vi "FPGA Beam Scanning beta.vi"(1 "Detectors":T1, 2 "Image Acquisition Parameters":T2={"Scan Type"=enum."Sample Scanning", "Scan Mode"=enum."XY", "Fast Axis Frequency (Hz)"=100.0, "Image Format"=128, "Line Accumulations"=1, "Frames Per Capture"=1, "Frames Accumulations"=1, "Image Dimension (um)"=[], "Number of Z Steps"=1, "Z Steps Size (um)"=1.0, "Pixel Size (nm)"=[]} {"Z Steps Size (um)" min=0.0; "Number of Z Steps" min=1; "Frames Accumulations" min=1; "Frames Per Capture" min=1; "Line Accumulations" min=1; "Image Format" items=["64 x 64"=64, "128 x 128"=128, "256 x 256"=256, "512 x 512"=512, "1024 x 1024"=1024, "2048 x 2048"=2048]}) -> ()   [LabVIEW 2016]
uses:
  <vilib>/rvi/interface/nirviReadWriteControl/nirviReadWriteControl.xnode
  <vilib>/rvi/interface/nirviMethod/nirviMethod.xnode
  <vilib>/rvi/errors/niLvFpgaMergeErrorWithErrorCode.vi
  <vilib>/rvi/interface/nirviOpenFPGA/nirviOpenFPGA.xnode
  <vilib>/vision/NI_Vision_Development_Module.lvlib
  <vilib>/rvi/interface/nirviCloseFPGA/nirviCloseFPGA.xnode
  <vilib>/vision/Image Controls.llb/IMAQ Image.ctl
  FPGA Bitfiles/MainSTEDFPGAProj_FPGATarget2_BeamScanningCamb_PyGckhW3v70.lvbitx
  FPGA Target VIs/FPGA-7852R/Beam Scanning Cambridge V1.vi
  Type Defs/Image Acquisition Parameters.ctl
  Detectors.ctl
panel:
  in  "line by line":bool
  in  "Adjust Trigger":u16=300
  # "Copyright (C) 2020 Edward S Allgeyer\n\nRedistribution and use in source and binary forms, with or without\nmodification, are permitted provided that the following conditions\nare met:\n\n1. Redistributions of source code must retain the above copyright\n   notice, this list of conditions and the following disclaimer.\n\n2. Redistributions in binary form must reproduce the above copyright\n   notice, this list of conditions and the following disclaimer in\n   the documentation and/or other materials provided with the\n   distribution.\n\n3. Neither the name of the copyright holder nor the names of its\n   contributors may be used to endorse or promote products derived\n   from this software without specific prior written permission.\n\nTHIS SOFTWARE IS PROVIDED BY THE COPYRIGHT HOLDERS AND CONTRIBUTORS\n\"AS IS\" AND ANY EXPRESS OR IMPLIED WARRANTIES, INCLUDING, BUT NOT\nLIMITED TO, THE IMPLIED WARRANTIES OF MERCHANTABILITY AND FITNESS\nFOR A PARTICULAR PURPOSE ARE DISCLAIMED. IN NO EVENT SHALL THE\nCOPYRIGHT HOLDER OR CONTRIBUTORS BE LIABLE FOR ANY DIRECT, INDIRECT,\nINCIDENTAL, SPECIAL, EXEMPLARY, OR CONSEQUENTIAL DAMAGES (INCLUDING,\nBUT NOT LIMITED TO, PROCUREMENT OF SUBSTITUTE GOODS OR SERVICES;\nLOSS OF USE, DATA, OR PROFITS; OR BUSINESS INTERRUPTION) HOWEVER\nCAUSED AND ON ANY THEORY OF LIABILITY, WHETHER IN CONTRACT, STRICT\nLIABILITY, OR TORT (INCLUDING NEGLIGENCE OR OTHERWISE) ARISING IN\nANY WAY OUT OF THE USE OF THIS SOFTWARE, EVEN IF ADVISED OF THE\nPOSSIBILITY OF SUCH DAMAGE."
  # "XY"
  # "Z"
  # "Length"
  # "Height"
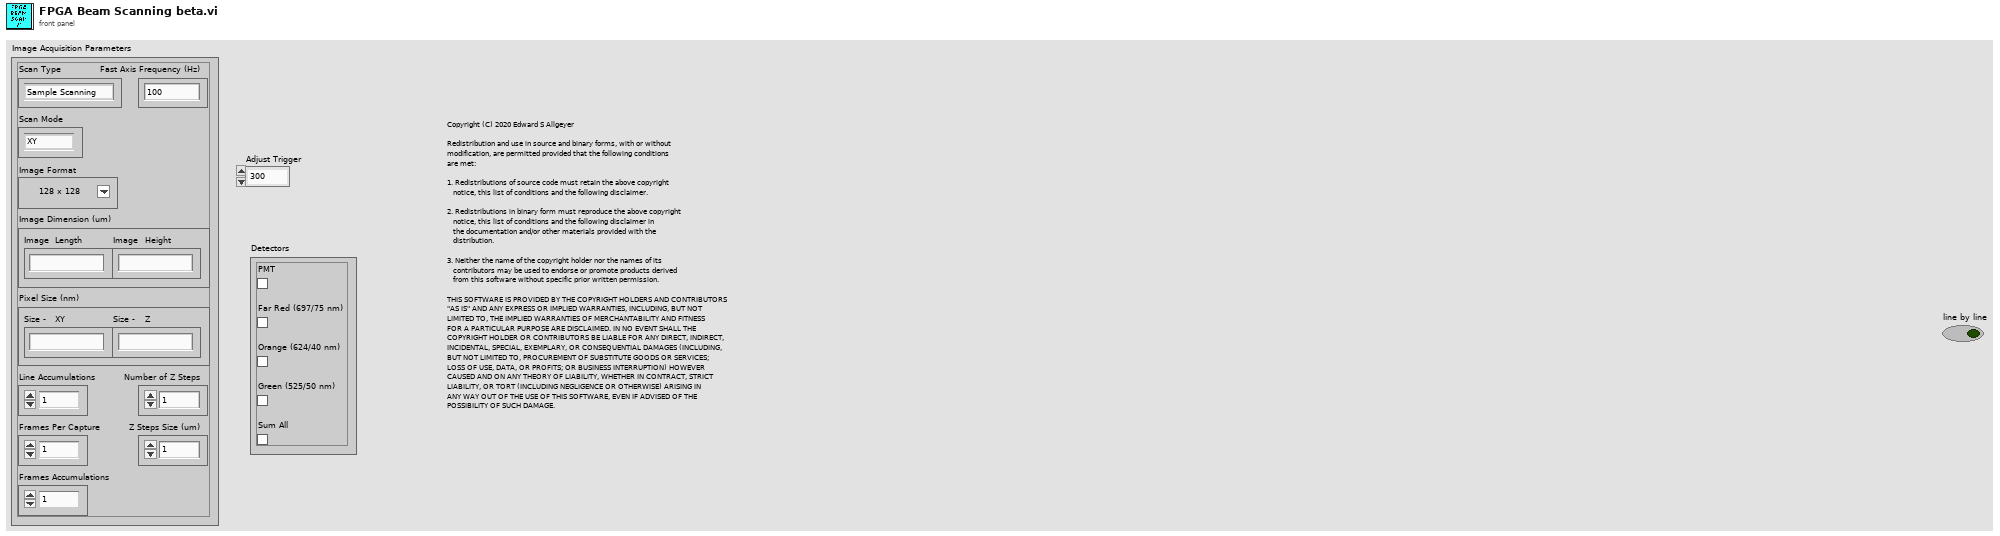
[diagram p1: front panel]
types:
  T1 = typedef "Detectors.ctl" = cluster{"PMT":bool, "Far Red (697/75 nm)":bool, "Orange (624/40 nm)":bool, "Green (525/50 nm)":bool, "Sum All":bool}
  T2 = typedef "Image Acquisition Parameters.ctl" = cluster{"Scan Type":enum16{"Sample Scanning", "Beam Scanning"}, "Scan Mode":enum16{"XY", "XZ", "YZ", "XYZ"}, "Fast Axis Frequency (Hz)":dbl, "Image Format":u16, "Line Accumulations":u16, "Frames Per Capture":u16, "Frames Accumulations":u16, "Image Dimension (um)":dbl[], "Number of Z Steps":u8, "Z Steps Size (um)":dbl, "Pixel Size (nm)":dbl[]}
  T3 = enum16{"big-endian, network order", "native, host order", "little-endian"}
  T4 = typedef "IMAQ Image.ctl" = refnum<image>
  T5 = cluster{"FPGA Sampling Period (ns)":dbl, "Counting Period (us)":dbl, "Samples Per Counting Period":i32, "Start Time (us)":dbl, "Stop Time (us)":dbl, "Normalized Scan End Position":dbl, "Normalized Scan Start Position":dbl}
  T6 = typedef "Scan Parameters.ctl" = cluster{"Fast_Ax_Amp_V":dbl, "Fast_Ax_Off_V":dbl, "Slow_Ax_Amp_V":dbl, "Slow_Ax_Off_V ":dbl, "Slow_Ax_Max_V_VperS":dbl, "Slow_Ax1_Del25ns":i32, "Slow_Ax2_Del25ns":i32, "Stage_X_Off_V":dbl, "Stage_Y_Off_V":dbl, "Stage_Z_Off_V":dbl, "Galvo1_Off_V":dbl, "Galvo2_Off_V":dbl, "Last_Scan_Mode":enum16{"XY", "XZ", "YZ", "XYZ"}, "Current_Scan_Mode":enum16{"XY", "XZ", "YZ", "XYZ"}, "Fly_Back_Lines":u16, "Linear_Ramp_End":u32, "Z_Step_I16":i16, "Z_Start_I16":i16, "Laser_States _U32":u32, "590_Voltage_I16":i16, "775_AOM_Volt_I16":i16, "Blanking OFF":bool, "Unused_Axis_I16":i16}
  T7 = typedef "Sequence Cluster_Ctrl.ctl" = cluster{"Image Acquisition Parameters":T2, "Laser Parameters":T8, "Detectors Parameters":T1, "Repeat":dbl, "LinebyLine":bool}
  T8 = typedef "Laser Controls.ctl" = cluster{"STED Power (0-5V)":dbl, "STED":bool, "640 nm":bool, "485 nm":bool, "Manual Control":bool, "White Light":bool, "405 nm":bool, "405 Power (0-5V)":dbl}
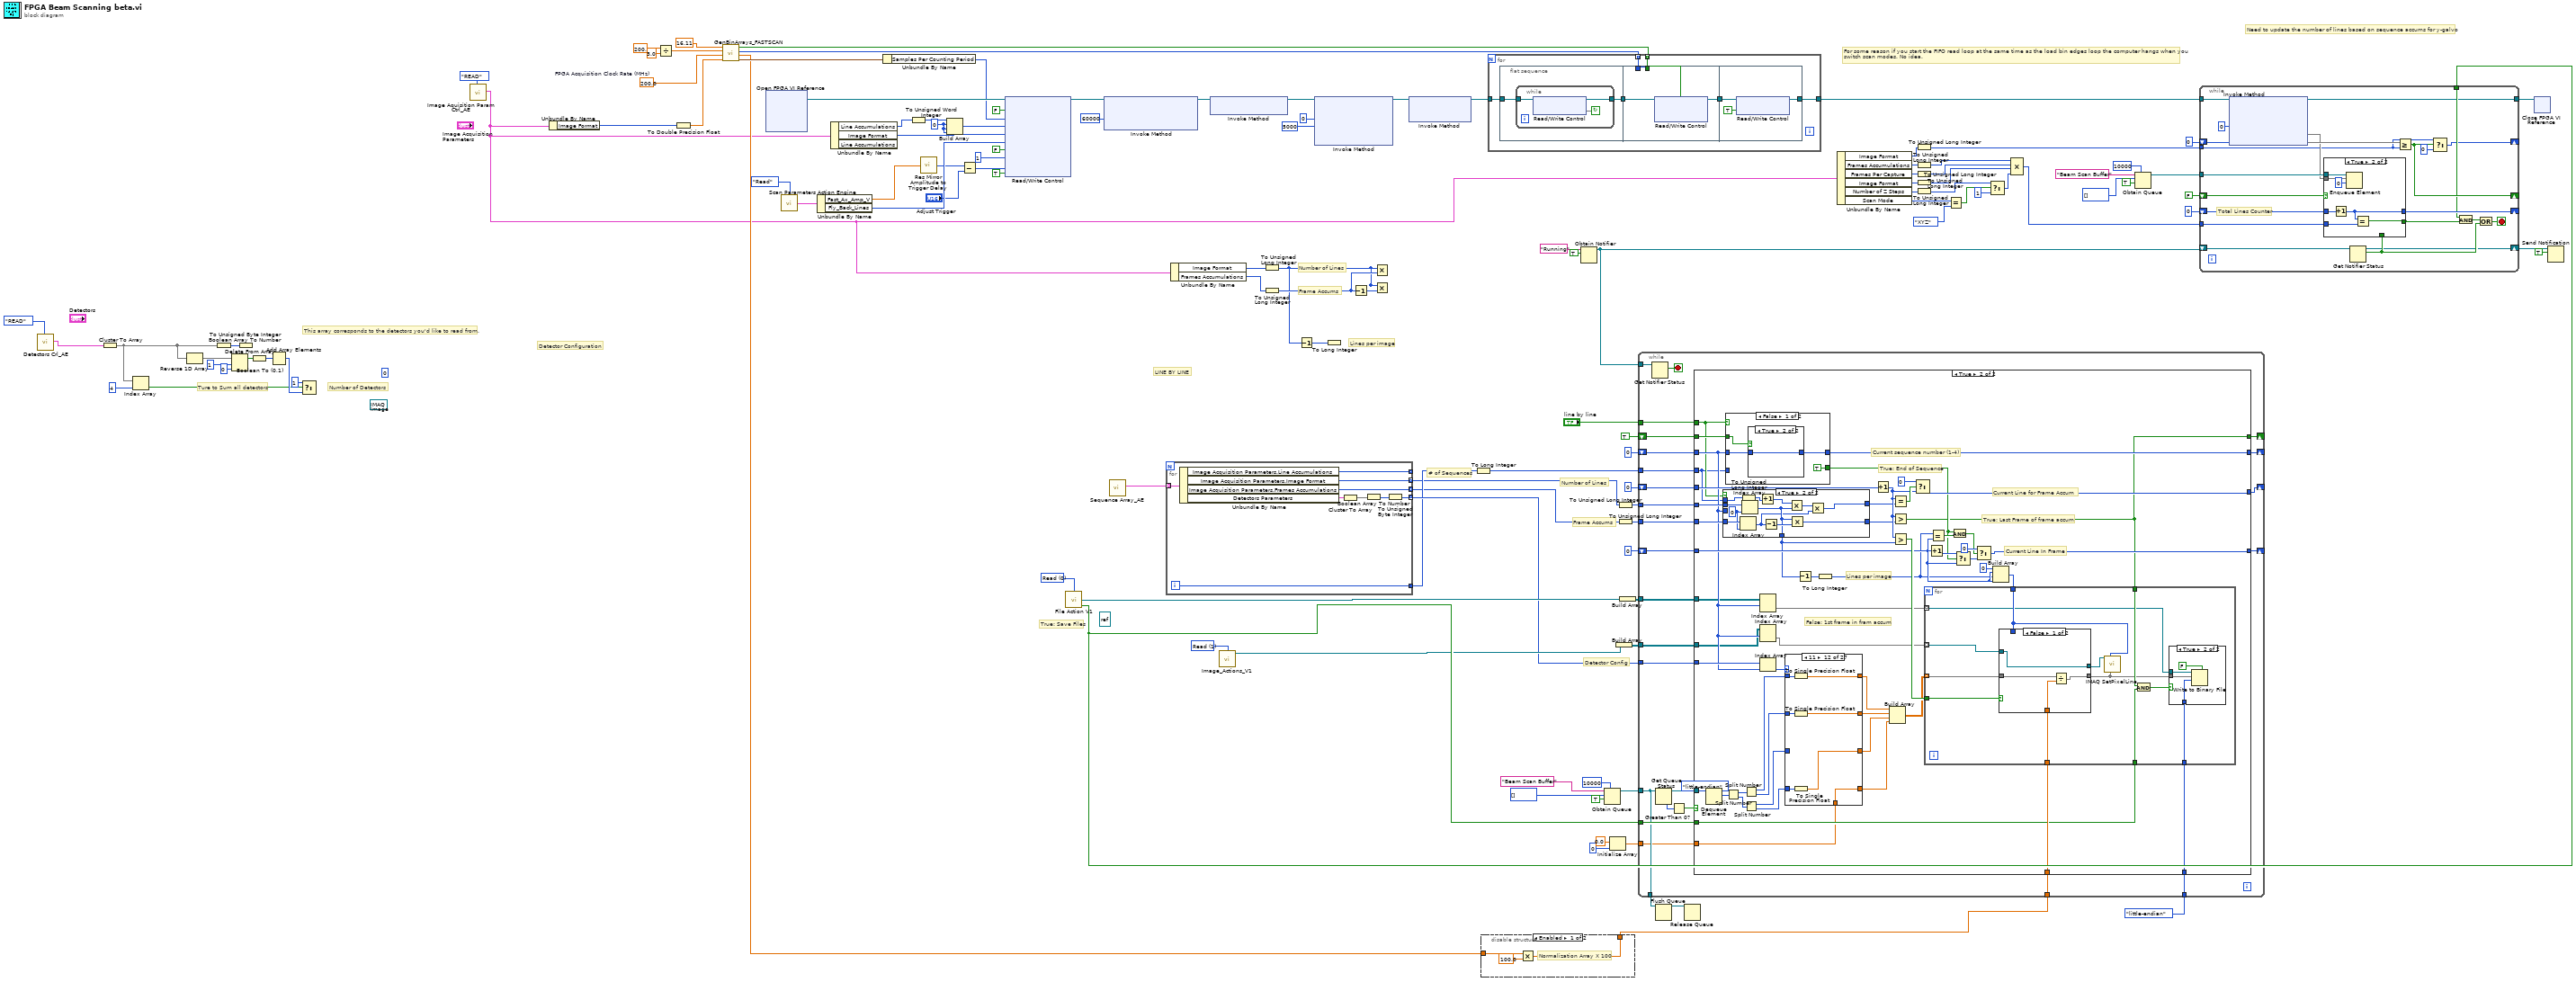
[diagram p0: block diagram]
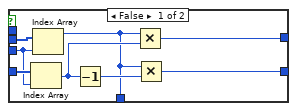
[diagram p3: hidden frame]
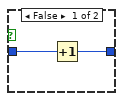
[diagram p4: hidden frame]
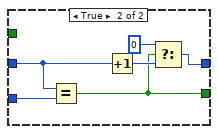
[diagram p5: hidden frame]
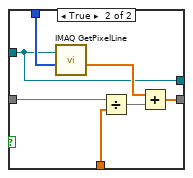
[diagram p7: hidden frame]
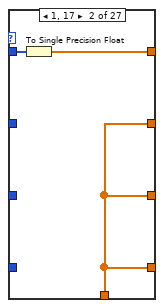
[diagram p9: hidden frame]
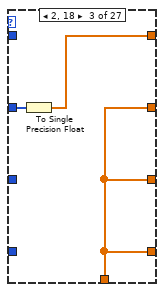
[diagram p10: hidden frame]
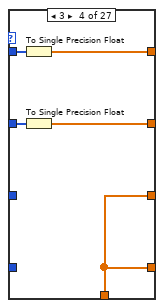
[diagram p11: hidden frame]
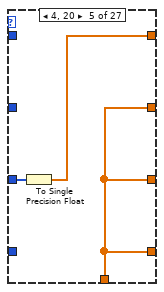
[diagram p12: hidden frame]
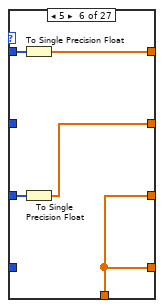
[diagram p13: hidden frame]
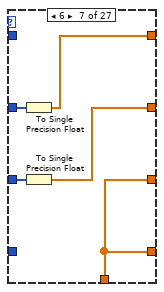
[diagram p14: hidden frame]
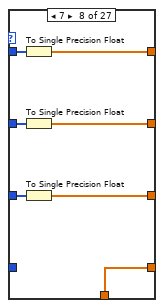
[diagram p15: hidden frame]
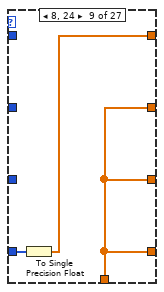
[diagram p16: hidden frame]
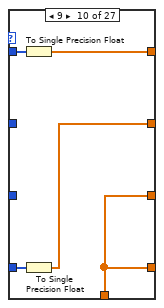
[diagram p17: hidden frame]
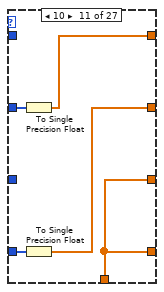
[diagram p18: hidden frame]
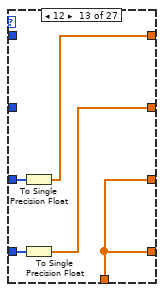
[diagram p19: hidden frame]
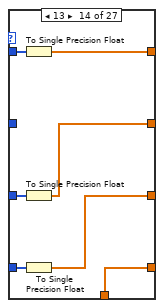
[diagram p20: hidden frame]
diagram:
  w48 = u16 0 items=["Read", "Write"] ("Mode")
  w49 = u16 0 ("element")
  (unwired) 0 ("Offset")
  w77 = refnum<file> refnum ("element")
  (unwired) T4 refnum ("New Image")
  w78 = u16 1 items=["Write", "Read"] ("Mode")
  (unwired) T3."little-endian" ("byte order (0:big-endian, network order)")
  w123 = 200.0  # FPGA Acquisition Clock Rate (MHz)
  # "# of Sequences"
  # "Detector Config"
  # "LINE BY LINE"
  # "Frame Accums"
  # "Number of Lines"
  # "This array corresponds to the detectors you'd like to read from."
  # "Ture to Sum all detectors"
  # "Number of Detectors"
  # "Detector Configuration"
  # "Frame Accums"
  # "Number of Lines"
  # "True: Save Files"
  # "Lines per image"
  # "For some reason if you start the FIFO read loop at the same time as the load bin edges loop the computer hangs when you\nswitch scan modes. No idea."
  # "Need to update the number of lines based on sequence accums for y-galvo"
  n1 = call "Detectors Crl_AE.vi"("Action"=enum16{"READ", "WRITE"}."READ") -> ("Detectors Parameters Out"=w32:T1)  [unwired: 10 in]
  n2 = Cluster To Array(cluster=w32) -> (array=w38:bool[])
  n3 = Index Array(array=w38, index=4) -> (element=w36:bool)
  n4 = Reverse 1D Array(array=w38) -> (reversed array=w72:bool[])
  n5 = Boolean Array To Number(Boolean array=w38) -> (number=w40:u32)
  n6 = Delete From Array(array=w72, length=1, index=0) -> (array with subset deleted=w76:bool[])  [unwired: 1 out]
  n7 = To Unsigned Byte Integer(number=w40) -> (unsigned 8bit integer=w39:u8)
  n8 = Boolean To (0,1)(Boolean=w76) -> (0, 1=w75:i16[])
  n9 = Add Array Elements(numeric array=w75) -> (sum=w74:i16)
  n10 = Select(t=i16 1, s=w36, f=w74) -> (s? t:f=w69:i16)
  n11 = call "Image Aquisition Param Ctrl_AE.vi"("Action"=enum16{"READ", "WRITE"}."READ") -> ("Image Acquisition Parameters Out"=w34:T2)  [unwired: 10 in]
  n12 = Unbundle By Name(w34) -> ("Image Format"=w47:u16)
  n13 = Divide(x=200.0, y=3.0) -> (x/y=w120:dbl)
  n14 = To Double Precision Float(number=w47) -> (double precision float=w104:dbl)
  n15 = call "GenBinArrays_FASTSCAN.vi"("Pixels Per Line"=w104, "FPGA Acquisition Clock Rate (MHz)"=w123, "Collection Percent (%)"=w120, "Scan Rate (kHz)"=16.11) -> ("Reported Parameters"=w119:T5, "Normalization Array"=w68:sgl[], "Pre Binned Counts (x100)"=w44:u32[], "FPGA Bin Edges"=w45:bool[])
  n16 = xnode "Open FPGA VI Reference"() -> ("FPGA VI Reference Out"=w127:refnum<k20>)  [unwired: 2 in, 1 out]
  n17 = call "Scan Parameters Action Engine.vi"("Action"=enum16{"Read", "Write"}."Read") -> ("Scan Parameters OUT"=w53:T6)  [unwired: 14 in]
  n18 = Unbundle By Name(w53) -> ("Fast_Ax_Amp_V"=w46:dbl, "Fly_Back_Lines"=w52:u16)
  n19 = Unbundle By Name(w34) -> ("Line Accumulations"=w58:u16, "Image Format"=w55:u16)  [unwired: 1 out]
  n20 = Unbundle By Name(w119) -> ("Samples Per Counting Period"=w87:i32)
  n21 = To Unsigned Word Integer(number=w58) -> (unsigned 16bit integer=w57:u16)
  n22 = call "Res Mirror Amplitude to Trigger Delay.vi"("Amplitude (V)"=w46) -> ("Trigger Delay (Ticks)"=w43:u16)
  n23 = Build Array(w57, w49, w49, w49) -> (w56:u16[])
  n24 = Subtract(x=w43, y="Adjust Trigger") -> (x-y=w42:u16)
  n25 = xnode "Read/Write Control"("FPGA VI Reference In"=w127, "Ready For Write"=FALSE, "FPGA Samples"=w87, "Accums Per Line"=w56, "Lines Per Image"=w55, "Dead Lines"=w52, "Line Trigger"=FALSE, "Sequences"=u8 1, "Trigger Delay (Ticks)"=w42, "Stop Acquisition"=TRUE) -> ("FPGA VI Reference Out"=w126:refnum<k20>)  [unwired: 1 in, 1 out]
  n26 = call "File Action V1.vi"("Mode"=w48) -> ("File REFs"=w29:refnum<file>[], "Files Open"=w28:bool)  [unwired: 12 in, 1 out]
  n27 = xnode "Invoke Method"("FPGA VI Reference In"=w126, "Requested Depth"=u32 60000) -> ("FPGA VI Reference Out"=w102:refnum<k20>)  [unwired: 1 in, 2 out]
  n28 = call "Sequence Array_AE.vi"() -> ("Sequence Cluster Array Out"=w26:T7[])  [unwired: 11 in]
  n29 = for {
    tunnel: w26 -> [w136] mode=indexing
    tunnel: [w135] -> w4 mode=indexing
    tunnel: [w134] -> w3 mode=indexing
    tunnel: [w133] -> _ mode=indexing
    tunnel: [w129] -> w25 mode=indexing
    tunnel: [w128] -> w6
    i -> [w128]
    n30 = Unbundle By Name(w136) -> ("Image Acquisition Parameters.Line Accumulations"=w133:u16, "Image Acquisition Parameters.Image Format"=w135:u16, "Image Acquisition Parameters.Frames Accumulations"=w134:u16, "Detectors Parameters"=w130:T1)
    n31 = Cluster To Array(cluster=w130) -> (array=w132:bool[])
    n32 = Boolean Array To Number(Boolean array=w132) -> (number=w131:u32)
    n33 = To Unsigned Byte Integer(number=w131) -> (unsigned 8bit integer=w129:u8)
  }
  n34 = Unbundle By Name(w34) -> ("Image Format"=w95:u16, "Frames Accumulations"=w94:u16)
  n35 = xnode "Invoke Method"("FPGA VI Reference In"=w102) -> ("FPGA VI Reference Out"=w103:refnum<k20>)  [unwired: 1 in, 1 out]
  n36 = call "Image_Actions_V1.vi"("Mode"=w78) -> ("Image REFs OUT"=w27:T4[])  [unwired: 13 in, 1 out]
  n37 = To Unsigned Long Integer(number=w95) -> (unsigned 32bit integer=w80:u32)
  n38 = To Unsigned Long Integer(number=w94) -> (unsigned 32bit integer=w81:u32)
  n39 = Decrement(x=w80) -> (x-1=w79:u32)
  n40 = xnode "Invoke Method"("FPGA VI Reference In"=w103, "Number of Elements"=u32 0, "Timeout (ms)"=5000) -> ("FPGA VI Reference Out"=w125:refnum<k20>)  [unwired: 1 in, 3 out]
  n41 = To Long Integer(number=w79) -> (32bit integer=w85:i32)
  n42 = Decrement(x=w81) -> (x-1=w84:u32)
  n43 = Multiply(x=w80, y=w81) -> (x*y=w82:u32)
  n44 = Multiply(x=w80, y=w84) -> (x*y=w83:u32)
  n45 = xnode "Invoke Method"("FPGA VI Reference In"=w125) -> ("FPGA VI Reference Out"=w118:refnum<k20>)  [unwired: 2 in, 1 out]
  n46 = To Long Integer(number=w6) -> (32bit integer=w5:i32)
  n47 = disable-structure shown="Enabled" {
    disable-tunnel: [w139 w140] -> w30
    disable-tunnel: w68 -> [w137 w143]
    frame Enabled {
      # "Normalization Array X 100"
      n48 = Multiply(x=w137, y=sgl 100.0) -> (x*y=w139:sgl[])
    }
    frame Disabled {
      n49 = Array Size(array=w143) -> (size(s)=w142:i32)
      n50 = Initialize Array(sgl 100.0 ("element"), w142) -> (w140:sgl[])
    }
  }
  n51 = for {
    tunnel: [w147] -> w92
    tunnel: w118 -> [w146]
    tunnel: w45 -> [w145] mode=indexing
    tunnel: w44 -> [w144] mode=indexing
    n52 = flat-sequence {
      tunnel: [w151] -> w149
      tunnel: w146 -> [w150]
      tunnel: w149 -> [w158]
      tunnel: [w157] -> w148
      tunnel: w145 -> [w156]
      tunnel: w144 -> [w155]
      tunnel: w148 -> [w161]
      tunnel: [w160] -> w147
      frame #0 {
        n53 = while {
          tunnel: [w154] -> w151
          tunnel: w150 -> [w153]
          stop <- w152 continue-if-true
          n54 = xnode "Read/Write Control"("FPGA VI Reference In"=w153) -> ("FPGA VI Reference Out"=w154:refnum<k20>, "Ready For Write"=w152)  [unwired: 1 in, 1 out]
        }
      }
      frame #1 {
        n55 = xnode "Read/Write Control"("FPGA VI Reference In"=w158, "BinEdge"=w156, "PreBinnedValue"=w155) -> ("FPGA VI Reference Out"=w157:refnum<k20>)  [unwired: 1 in, 1 out]
      }
      frame #2 {
        n56 = xnode "Read/Write Control"("FPGA VI Reference In"=w161, "Ready For Write"=TRUE) -> ("FPGA VI Reference Out"=w160:refnum<k20>)  [unwired: 1 in, 1 out]
      }
    }
  }
  n57 = Obtain Notifier(name (unnamed)="Running", notification data type=TRUE) -> (notifier out=w31:refnum<notifier>)  [unwired: 2 in, 2 out]
  n58 = Obtain Queue(max queue size (-1, unlimited)=10000, name (unnamed)="Beam Scan Buffer", element data type=u64[] [], create if not found? (T)=TRUE) -> (queue out=w23:refnum<queue>)  [unwired: 1 in, 2 out]
  n59 = Initialize Array(sgl 0.0, 0 ("dimension size")) -> (w12:sgl[])
  n60 = Build Array(w27) -> (w7:T4[][])
  n61 = To Unsigned Long Integer(number=w3) -> (unsigned 32bit integer=w1:u32[])
  n62 = To Unsigned Long Integer(number=w4) -> (unsigned 32bit integer=w2:u32[])
  n63 = Build Array(w29) -> (w8:refnum<file>[][])
  n64 = while {
    shift-right: [w185] -> _
    shift-left: 0 -> [w186]
    tunnel: T3."little-endian" ("byte order (0:big-endian, network order)") -> [w184]
    tunnel: w30 -> [w183]
    tunnel: w28 -> [w182]
    tunnel: w31 -> [w178]
    shift-right: [w175] -> _
    shift-left: u32 0 -> [w176]
    tunnel: w1 -> [w174]
    tunnel: w2 -> [w173]
    tunnel: w23 -> [w172]
    tunnel: [w172] -> w15
    tunnel: w12 -> [w171]
    tunnel: w7 -> [w170]
    tunnel: w8 -> [w169]
    tunnel: w25 -> [w168]
    shift-right: [w166] -> _
    shift-left: 0 -> [w167]
    tunnel: w5 -> [w165]
    tunnel: "line by line" -> [w164]
    shift-right: [w162] -> _
    shift-left: TRUE -> [w163]
    stop <- w177 stop-if-true
    n65 = Get Notifier Status(notifier=w178) -> (current notification=w177:bool)  [unwired: 1 in, 4 out]
    n66 = Get Queue Status(queue=w172) -> (queue out=w179:refnum<queue>, # elements in queue=w181:i32)  [unwired: 2 in, 6 out]
    n67 = Greater Than 0?(x=w181) -> (x > 0?=w180:bool)
    n68 = case shown="True" w180 {
      tunnel: w186 -> [w190 w213]
      tunnel: [w190 w237] -> w185
      tunnel: w184 -> [_ w236]
      tunnel: w183 -> [_ w235]
      tunnel: w182 -> [_ w227]
      tunnel: w179 -> [_ w234]
      tunnel: w176 -> [w189 w231]
      tunnel: [w189 w230] -> w175
      tunnel: w174 -> [_ w229]
      tunnel: w173 -> [_ w228]
      tunnel: w171 -> [_ w220]
      tunnel: w170 -> [_ w197]
      tunnel: w169 -> [_ w199]
      tunnel: w168 -> [_ w217]
      tunnel: w167 -> [w188 w200]
      tunnel: [w188 w216] -> w166
      tunnel: w165 -> [_ w192]
      tunnel: w164 -> [_ w195]
      tunnel: w163 -> [w187 w204]
      tunnel: [w187 w203] -> w162
      frame False {
      }
      frame True {
        # "Lines per image"
        # "True: End of Sequence"
        # "Current sequence number (1-4)"
        # "False: 1st frame in fram accum"
        # "True: Last Frame of frame accum"
        # "Current Line for Frame Accum"
        # "Current Line In Frame"
        n69 = Dequeue Element(queue=w234) -> (element=w241:u64[])  [unwired: 2 in, 3 out]
        n70 = case shown="True" w195 {
          tunnel: w229 -> [w250 w262]
          tunnel: w228 -> [w249 w261]
          tunnel: [w246 w254] -> w202
          tunnel: [w244 w259] -> w201
          tunnel: w200 -> [w248 _]
          tunnel: [w243 w258] -> w191
          tunnel: w192 -> [_ w256]
          frame False {
            n71 = Index Array(array=w250, index=w248) -> (element=w247:u32)
            n72 = Index Array(array=w249, index=w248) -> (element=w243:u32)
            n73 = Decrement(x=w247) -> (x-1=w245:u32)
            n74 = Multiply(x=w243, y=w247) -> (x*y=w246:u32)
            n75 = Multiply(x=w243, y=w245) -> (x*y=w244:u32)
          }
          frame True {
            w257 = 0
            n76 = Index Array(array=w262, index=w257) -> (element=w252:u32)
            n77 = To Unsigned Long Integer(number=w256) -> (unsigned 32bit integer=w251:u32)
            n78 = Index Array(array=w261, index=w257) -> (element=w258:u32)
            n79 = Increment(x=w251) -> (x+1=w255:u32)
            n80 = Decrement(x=w252) -> (x-1=w260:u32)
            n81 = Multiply(x=w255, y=w258) -> (x*y=w253:u32)
            n82 = Multiply(x=w258, y=w260) -> (x*y=w259:u32)
            n83 = Multiply(x=w253, y=w252) -> (x*y=w254:u32)
          }
        }
        n84 = case shown="False" w195 {
          tunnel: [w266 w273] -> w216
          tunnel: w192 -> [_ w272]
          tunnel: w200 -> [w265 w271]
          tunnel: [TRUE w270] -> w211
          tunnel: w204 -> [w264 _]
          frame False {
            n85 = case shown="True" w264 {
              tunnel: [w267 w269] -> w266
              tunnel: w265 -> [w268 w269]
              frame False {
                n86 = Increment(x=w268) -> (x+1=w267:i32)
              }
              frame True {
              }
            }
          }
          frame True {
            n87 = Equal?(x=w271, y=w272) -> (x = y?=w270:bool)
            n88 = Increment(x=w271) -> (x+1=w275:i32)
            n89 = Select(t=0, s=w270, f=w275) -> (s? t:f=w273:i32)
          }
        }
        n90 = Split Number(x=w241) -> (hi(x)=w242:u32[], lo(x)=w240:u32[])
        n91 = Split Number(x=w242) -> (hi(x)=w224:u16[], lo(x)=w223:u16[])
        n92 = Split Number(x=w240) -> (hi(x)=w222:u16[], lo(x)=w221:u16[])
        n93 = Index Array(array=w199, index (row)=w200) -> (element=w198:refnum<file>[])  [unwired: 1 in]
        n94 = Index Array(array=w197, index (row)=w200) -> (element=w196:T4[])  [unwired: 1 in]
        n95 = Index Array(array=w217, index=w200) -> (element=w218:u8)
        n96 = case shown="11" w218 {
          tunnel: w224 -> [_ w306 _ w313 _ w322 _ w334 _ w342 _ w354 _ w366 _ w381 w386 w393 _ w407 w413 _ w427 _ w441 _ w459]
          tunnel: w223 -> [_ _ w309 w314 _ _ w327 w333 _ _ w347 w353 _ _ w373 w380 w387 _ w399 w406 _ w419 w426 _ _ w449 w458]
          tunnel: w222 -> [_ _ _ _ w317 w321 w326 w332 _ _ _ _ w359 w365 w372 w379 _ w392 w398 w405 _ _ _ w433 w440 w448 w457]
          tunnel: w221 -> [_ _ _ _ _ _ _ _ w337 w341 w346 w352 w358 w364 w371 w378 _ _ _ _ w412 w418 w425 w432 w439 w447 w456]
          tunnel: [w303 w305 w308 w312 w316 w320 w325 w331 w336 w340 w345 w351 w357 w363 w370 w377 w384 w389 w396 w401 w409 w417 w423 w431 w435 w446 w455] -> w208
          tunnel: [w303 w304 w307 w311 w315 w319 w324 w330 w335 w339 w344 w350 w356 w362 w369 w376 w382 w388 w394 w400 w408 w414 w420 w428 w434 w442 w450] -> w209
          tunnel: [w303 w304 w307 w310 w315 w318 w323 w329 w335 w338 w343 w349 w355 w361 w368 w375 w382 w388 w394 w400 w408 w414 w420 w428 w434 w442 w450] -> w207
          tunnel: [w303 w304 w307 w310 w315 w318 w323 w328 w335 w338 w343 w348 w355 w360 w367 w374 w382 w388 w394 w400 w408 w414 w420 w428 w434 w442 w450] -> w206
          tunnel: w220 -> [w303 w304 w307 w310 w315 w318 w323 w328 w335 w338 w343 w348 w355 w360 w367 _ w382 w388 w394 w400 w408 w414 w420 w428 w434 w442 w450]
          frame 0, 16, Default {
          }
          frame 1, 17 {
            n97 = To Single Precision Float(number=w306) -> (single precision float=w305:sgl[])
          }
          frame 2, 18 {
            n98 = To Single Precision Float(number=w309) -> (single precision float=w308:sgl[])
          }
          frame 3 {
            n99 = To Single Precision Float(number=w313) -> (single precision float=w312:sgl[])
            n100 = To Single Precision Float(number=w314) -> (single precision float=w311:sgl[])
          }
          frame 4, 20 {
            n101 = To Single Precision Float(number=w317) -> (single precision float=w316:sgl[])
          }
          frame 5 {
            n102 = To Single Precision Float(number=w322) -> (single precision float=w320:sgl[])
            n103 = To Single Precision Float(number=w321) -> (single precision float=w319:sgl[])
          }
          frame 6 {
            n104 = To Single Precision Float(number=w327) -> (single precision float=w325:sgl[])
            n105 = To Single Precision Float(number=w326) -> (single precision float=w324:sgl[])
          }
          frame 7 {
            n106 = To Single Precision Float(number=w334) -> (single precision float=w331:sgl[])
            n107 = To Single Precision Float(number=w333) -> (single precision float=w330:sgl[])
            n108 = To Single Precision Float(number=w332) -> (single precision float=w329:sgl[])
          }
          frame 8, 24 {
            n109 = To Single Precision Float(number=w337) -> (single precision float=w336:sgl[])
          }
          frame 9 {
            n110 = To Single Precision Float(number=w342) -> (single precision float=w340:sgl[])
            n111 = To Single Precision Float(number=w341) -> (single precision float=w339:sgl[])
          }
          frame 10 {
            n112 = To Single Precision Float(number=w347) -> (single precision float=w345:sgl[])
            n113 = To Single Precision Float(number=w346) -> (single precision float=w344:sgl[])
          }
          frame 11 {
            n114 = To Single Precision Float(number=w354) -> (single precision float=w351:sgl[])
            n115 = To Single Precision Float(number=w353) -> (single precision float=w350:sgl[])
            n116 = To Single Precision Float(number=w352) -> (single precision float=w349:sgl[])
          }
          frame 12 {
            n117 = To Single Precision Float(number=w359) -> (single precision float=w357:sgl[])
            n118 = To Single Precision Float(number=w358) -> (single precision float=w356:sgl[])
          }
          frame 13 {
            n119 = To Single Precision Float(number=w366) -> (single precision float=w363:sgl[])
            n120 = To Single Precision Float(number=w365) -> (single precision float=w362:sgl[])
            n121 = To Single Precision Float(number=w364) -> (single precision float=w361:sgl[])
          }
          frame 14 {
            n122 = To Single Precision Float(number=w373) -> (single precision float=w370:sgl[])
            n123 = To Single Precision Float(number=w372) -> (single precision float=w369:sgl[])
            n124 = To Single Precision Float(number=w371) -> (single precision float=w368:sgl[])
          }
          frame 15 {
            n125 = To Single Precision Float(number=w381) -> (single precision float=w377:sgl[])
            n126 = To Single Precision Float(number=w380) -> (single precision float=w376:sgl[])
            n127 = To Single Precision Float(number=w379) -> (single precision float=w375:sgl[])
            n128 = To Single Precision Float(number=w378) -> (single precision float=w374:sgl[])
          }
          frame 19 {
            n129 = To Single Precision Float(number=w386) -> (single precision float=w385:sgl[])
            n130 = To Single Precision Float(number=w387) -> (single precision float=w383:sgl[])
            n131 = Add(x=w385, y=w383) -> (x+y=w384:sgl[])
          }
          frame 21 {
            n132 = To Single Precision Float(number=w393) -> (single precision float=w391:sgl[])
            n133 = To Single Precision Float(number=w392) -> (single precision float=w390:sgl[])
            n134 = Add(x=w391, y=w390) -> (x+y=w389:sgl[])
          }
          frame 22 {
            n135 = To Single Precision Float(number=w399) -> (single precision float=w397:sgl[])
            n136 = To Single Precision Float(number=w398) -> (single precision float=w395:sgl[])
            n137 = Add(x=w397, y=w395) -> (x+y=w396:sgl[])
          }
          frame 23 {
            n138 = To Single Precision Float(number=w407) -> (single precision float=w404:sgl[])
            n139 = To Single Precision Float(number=w406) -> (single precision float=w403:sgl[])
            n140 = To Single Precision Float(number=w405) -> (single precision float=w402:sgl[])
            n141 = Compound Arithmetic op=ADD(w404, w403, w402) -> (w401:sgl[])
          }
          frame 25 {
            n142 = To Single Precision Float(number=w413) -> (single precision float=w411:sgl[])
            n143 = To Single Precision Float(number=w412) -> (single precision float=w410:sgl[])
            n144 = Add(x=w411, y=w410) -> (x+y=w409:sgl[])
          }
          frame 26 {
            n145 = To Single Precision Float(number=w419) -> (single precision float=w416:sgl[])
            n146 = To Single Precision Float(number=w418) -> (single precision float=w415:sgl[])
            n147 = Add(x=w416, y=w415) -> (x+y=w417:sgl[])
          }
          frame 27 {
            n148 = To Single Precision Float(number=w427) -> (single precision float=w424:sgl[])
            n149 = To Single Precision Float(number=w426) -> (single precision float=w422:sgl[])
            n150 = To Single Precision Float(number=w425) -> (single precision float=w421:sgl[])
            n151 = Compound Arithmetic op=ADD(w424, w422, w421) -> (w423:sgl[])
          }
          frame 28 {
            n152 = To Single Precision Float(number=w433) -> (single precision float=w430:sgl[])
            n153 = To Single Precision Float(number=w432) -> (single precision float=w429:sgl[])
            n154 = Add(x=w430, y=w429) -> (x+y=w431:sgl[])
          }
          frame 29 {
            n155 = To Single Precision Float(number=w441) -> (single precision float=w438:sgl[])
            n156 = To Single Precision Float(number=w440) -> (single precision float=w437:sgl[])
            n157 = To Single Precision Float(number=w439) -> (single precision float=w436:sgl[])
            n158 = Compound Arithmetic op=ADD(w438, w437, w436) -> (w435:sgl[])
          }
          frame 30 {
            n159 = To Single Precision Float(number=w449) -> (single precision float=w445:sgl[])
            n160 = To Single Precision Float(number=w448) -> (single precision float=w444:sgl[])
            n161 = To Single Precision Float(number=w447) -> (single precision float=w443:sgl[])
            n162 = Compound Arithmetic op=ADD(w445, w444, w443) -> (w446:sgl[])
          }
          frame 31 {
            n163 = To Single Precision Float(number=w459) -> (single precision float=w454:sgl[])
            n164 = To Single Precision Float(number=w458) -> (single precision float=w453:sgl[])
            n165 = To Single Precision Float(number=w457) -> (single precision float=w452:sgl[])
            n166 = To Single Precision Float(number=w456) -> (single precision float=w451:sgl[])
            n167 = Compound Arithmetic op=ADD(w454, w453, w452, w451) -> (w455:sgl[])
          }
        }
        n168 = Decrement(x=w191) -> (x-1=w194:u32)
        n169 = To Long Integer(number=w194) -> (32bit integer=w193:i32)
        n170 = Increment(x=w231) -> (x+1=w226:u32)
        n171 = Build Array(w208, w209, w207, w206) -> (w205:sgl[][])
        n172 = Equal?(x=w226, y=w202) -> (x = y?=w233:bool)
        n173 = Greater?(x=w226, y=w201) -> (0:w203:bool)
        n174 = Greater?(x=w226, y=w191) -> (0:w225:bool)
        n175 = Select(t=u32 0, s=w233, f=w226) -> (s? t:f=w230:u32)
        n176 = Increment(x=w213) -> (x+1=w215:i32)
        n177 = Equal?(x=w193, y=w213) -> (x = y?=w212:bool)
        n178 = And(x=w211, y=w212) -> (x .and. y?=w210:bool)
        n179 = Select(t=w215, s=w211, f=w213) -> (s? t:f=w214:i32)
        n180 = Select(t=0, s=w210, f=w214) -> (s? t:f=w237:i32)
        n181 = Build Array(0, w213, w193, w213) -> (w219:i32[])
        n182 = for {
          tunnel: w236 -> [w287]
          tunnel: w235 -> [w286]
          tunnel: w203 -> [w285]
          tunnel: w227 -> [w284]
          tunnel: w225 -> [w283]
          tunnel: w205 -> [w282] mode=indexing
          tunnel: w219 -> [w281]
          tunnel: w196 -> [w276] mode=indexing
          tunnel: w198 -> [w277] mode=indexing
          n183 = case shown="False" w283 {
            tunnel: w282 -> [w292 w296]
            tunnel: [w295 w301] -> w280
            tunnel: w281 -> [_ w299]
            tunnel: w286 -> [w294 w298]
            tunnel: w276 -> [w293 w297]
            tunnel: [w293 w297] -> w278
            frame False {
              n184 = Divide(x=w292, y=w294) -> (x/y=w295:sgl[])
            }
            frame True {
              n185 = call "IMAQ GetPixelLine"("Line Coordinates"=w299, "Image"=w297) -> ("Pixels Line (Float)"=w300:sgl[])  [unwired: 2 in, 4 out]
              n186 = Divide(x=w296, y=w298) -> (x/y=w302:sgl[])
              n187 = Add(x=w300, y=w302) -> (x+y=w301:sgl[])
            }
          }
          n188 = call "IMAQ SetPixelLine"("Pixels Line (Float)"=w280, "Line Coordinates"=w281, "Image"=w278) -> ()  [unwired: 7 in, 2 out]
          n189 = And(x=w285, y=w284) -> (x .and. y?=w279:bool)
          n190 = case shown="True" w279 {
            tunnel: w280 -> [_ w291]
            tunnel: w287 -> [_ w289]
            tunnel: w277 -> [_ w288]
            frame False {
            }
            frame True {
              n191 = Write to Binary File(file (use dialog)=w288, data=w291, 5:FALSE ("prepend array or string size? (T)"), 9:w289) -> ()  [unwired: 2 in, 3 out]
            }
          }
        }
      }
    }
  }
  n192 = Flush Queue(queue=w15) -> (queue out=w22:refnum<queue>)  [unwired: 1 in, 2 out]
  n193 = Release Queue(queue=w22) -> ()  [unwired: 2 in, 3 out]
  n194 = Unbundle By Name(w34) -> ("Image Format"=w110:u16, "Frames Accumulations"=w66:u16, "Frames Per Capture"=w111:u16, "Image Format"=w67:u16, "Number of Z Steps"=w63:u8, "Scan Mode"=w64:enum16{"XY", "XZ", "YZ", "XYZ"})
  n195 = To Unsigned Long Integer(number=w110) -> (unsigned 32bit integer=w117:u32)
  n196 = To Unsigned Long Integer(number=w66) -> (unsigned 32bit integer=w62:u32)
  n197 = To Unsigned Long Integer(number=w111) -> (unsigned 32bit integer=w61:u32)
  n198 = To Unsigned Long Integer(number=w67) -> (unsigned 32bit integer=w60:u32)
  n199 = To Unsigned Long Integer(number=w63) -> (unsigned 32bit integer=w59:u32)
  n200 = Equal?(x=w64, y=enum16{"XY", "XZ", "YZ", "XYZ"}."XYZ") -> (x = y?=w98:bool)
  n201 = Select(t=w59, s=w98, f=u32 1) -> (s? t:f=w97:u32)
  n202 = Compound Arithmetic op=MULTIPLY(w62, w61, w60, w97) -> (w112:u32)
  n203 = Obtain Queue(max queue size (-1, unlimited)=10000, name (unnamed)="Beam Scan Buffer", element data type=u64[] [], create if not found? (T)=TRUE) -> (queue out=w50:refnum<queue>)  [unwired: 1 in, 2 out]
  n204 = while {
    tunnel: w92 -> [w480]
    shift-right: [w462] -> _
    shift-left: u32 0 -> [w461]
    tunnel: w117 -> [w460]
    shift-right: [w476] -> _
    shift-left: FALSE -> [w475]
    tunnel: w50 -> [w474]
    shift-right: [w472] -> _
    shift-left: u32 0 -> [w473]
    tunnel: w112 -> [w468]
    tunnel: w28 -> [w465]
    tunnel: [w463] -> w93
    shift-right: [w464] -> w106
    shift-left: w31 -> [w481]
    stop <- w471 stop-if-true
    # "Total Lines Counter"
    n205 = xnode "Invoke Method"("FPGA VI Reference In"=w480, "Number of Elements"=w461, "Timeout (ms)"=0) -> ("FPGA VI Reference Out"=w463:refnum<k20>, "Data"=w469:void[], "Elements Remaining"=w478)  [unwired: 1 in, 1 out]
    n206 = Get Notifier Status(notifier=w481) -> (notifier out=w464:refnum<notifier>, current notification=w470:bool)  [unwired: 1 in, 3 out]
    n207 = case shown="True" w475 {
      tunnel: w469 -> [_ w484]
      tunnel: w474 -> [_ w490]
      tunnel: w473 -> [w483 w487]
      tunnel: [w483 w488] -> w472
      tunnel: [w482 w486] -> w467
      tunnel: w470 -> [w482 _]
      tunnel: w468 -> [_ w485]
      frame False {
      }
      frame True {
        n208 = Increment(x=w487) -> (x+1=w488:u32)
        n209 = Enqueue Element(queue=w490, element=w484, timeout in ms (-1)=0) -> ()  [unwired: 1 in, 3 out]
        n210 = Equal?(x=w488, y=w485) -> (x = y?=w486:bool)
      }
    }
    n211 = Greater Or Equal?(x=w478, y=w460) -> (x >= y?=w476:bool)
    n212 = Select(t=w460, s=w476, f=u32 0) -> (s? t:f=w462:u32)
    n213 = And(x=w465, y=w467) -> (x .and. y?=w466:bool)
    n214 = Or(x=w466, y=w470) -> (x .or. y?=w471:bool)
  }
  n215 = xnode "Close FPGA VI Reference"("FPGA VI Reference In"=w93) -> ()  [unwired: 1 in, 1 out]
  n216 = Send Notification(notification=TRUE, notifier=w106) -> ()  [unwired: 1 in, 2 out]
